vi "Clean Up.vi"(8 "error in":errorcluster, 11 "pipe in":T1) -> (0 "error out":errorcluster)   [LabVIEW 2019, in "LV Process library.lvlib"]
doc: "Calls lv_proc.dll to close process instance handle (part of pipe handle). This VI does not terminates the process, only closes opened handles. It is required to be called after the process returnes exit code otherwise all handles (process, main thread, pipes) stays opened.\n\n---\nLV Process works only with lv_proc.dll library, which is part of vipm package or should be delivered together with packed library. Placement of this dll is selected in terminal of Create Process.vi."
uses:
  LV Process library.lvlib
  Pipe Handle.ctl
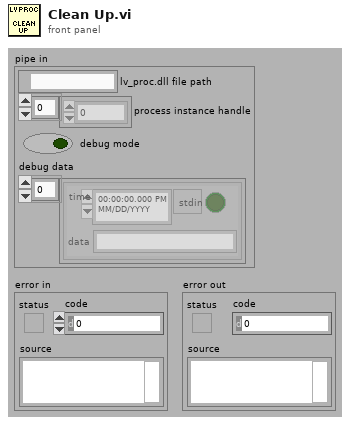
[diagram p1: front panel]
types:
  T1 = typedef "LV Process library.lvlib/Pipe Handle.ctl" = cluster{"lv_proc.dll file path":path, "process instance handle":u32[], "debug mode":bool, "debug data":cluster{"time":timestamp, "stdin":bool, "data":string}[]}
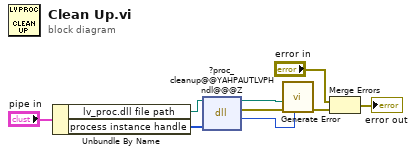
[diagram p0: block diagram]
diagram:
  n1 = Unbundle By Name("pipe in") -> ("lv_proc.dll file path"=w8:path, "process instance handle"=w7:u32[])
  n2 = dll-call lib="C:/Data/GOLPI/LV Process/lv_proc.dll" fn="?proc_cleanup@@YAHPAUTLVPHndl@@@Z" label="proc_cleanup"(path in=w8, "proc"=w7) -> (path out=w3:path, error out=w2:errorcluster, "error"=w6:i32)  [unwired: 3 in]
  n3 = call "Generate Error.vi"("error code in"=w6, "error in"=w2, "lv_proc.dll path in"=w3) -> ("error out"=w1:errorcluster)  [unwired: 6 in, 1 out]
  n4 = Merge Errors("error in", w1) -> (→"error out":errorcluster)
